vi "assignment4.vi"() -> ()   [LabVIEW 2020]
panel:
  in  "Lower Cut-Off":dbl=30.0
  out "-3db  point":dbl=29.59150674433556
  out "XY Graph":cluster{i32, dbl}[](graph)=[{0, -3.0576747821188574e-08}, {1, -6.013728431780247e-07}, {2, -4.387539160816041e-06}, {3, 3.5095275010031514e-05}, {4, -9.967196479561105e-05}, {5, -0.0002790200036056059}, {6, 0.0011235149369299283}, {7, 0.001968581295715452}, {8, 0.000646352615420884}, {9, -0.0035665225984870207}, {10, -0.010539479788425375}, {11, -0.017748779017499362}, {12, -0.028426417413518115}, {13, -0.044156999314381426}, {14, -0.06675516657396055}, {15, -0.09841418213321976}, {16, -0.14139245078033086}, {17, -0.19793797481989572}, {18, -0.27157149734632635}, {19, -0.36557922218263733}, {20, -0.4489491833896813}, {21, -0.5558693293864396}, {22, -0.7148632709887328}, {23, -0.9010359791461806}, {24, -1.1179952654437506}, {25, -1.3703953898872534}, {26, -1.6597556218137142}, {27, -1.9858590320404002}, {28, -2.348495319765153}, {29, -2.745860990601728}, {30, -3.1755078405015484}, {31, -3.6338601009569373}, {32, -4.117814928392555}, {33, -4.623162452023611}, {34, -5.146444624309847}, {35, -5.683763470785429}, {36, -6.23144744610925}, {37, -6.786719315566659}, {38, -7.346502587344456}, {39, -7.90842063335817}, {40, -8.470649778077558}, {41, -9.03113712355663}, {42, -9.588761700267254}, {43, -10.134599451716804}, {44, -10.67333872530238}, {45, -11.206703608600378}, {46, -11.733812394204042}, {47, -12.252397753569275}, {48, -12.762929323776763}, {49, -13.266641370261848}]
  in  "frequency start":i32
  in  "frequency end":i32=50
  out "?":dynamicdata(graph)=[{"t0"=timestamp(3 s since 1904-01-01), "dt"=0.0001, "Y"=array[1000 elements], "attributes"=variant("NI_ChannelName"=variant(string "Sine_input"), "NI_ExpIsRelativeTime"=variant(bool TRUE), "NI_ExpStartTimeStamp"=variant(timestamp timestamp(3675059466.168606 s since 1904-01-01)), "NI_ExpTimeStamp"=variant(timestamp timestamp(3675059469.168606 s since 1904-01-01)), "NI_ExpXDimension"=variant(string "t"))}]
  in  "stop":bool
  out "Waveform Chart 2":dynamicdata(graph)=[{"t0"=timestamp(3 s since 1904-01-01), "dt"=0.0001, "Y"=array[1000 elements], "attributes"=variant("NI_ChannelName"=variant(string "Sine_input (Filtered)"), "NI_ExpIsRelativeTime"=variant(bool TRUE), "NI_ExpStartTimeStamp"=variant(timestamp timestamp(3675059466.168606 s since 1904-01-01)), "NI_ExpTimeStamp"=variant(timestamp timestamp(3675059469.168606 s since 1904-01-01)), "NI_ExpXDimension"=variant(string "t"), "NI_OriginalChannelName"=variant(string "Sine_input"))}]
  in  "Signal frequency":dbl=30.0
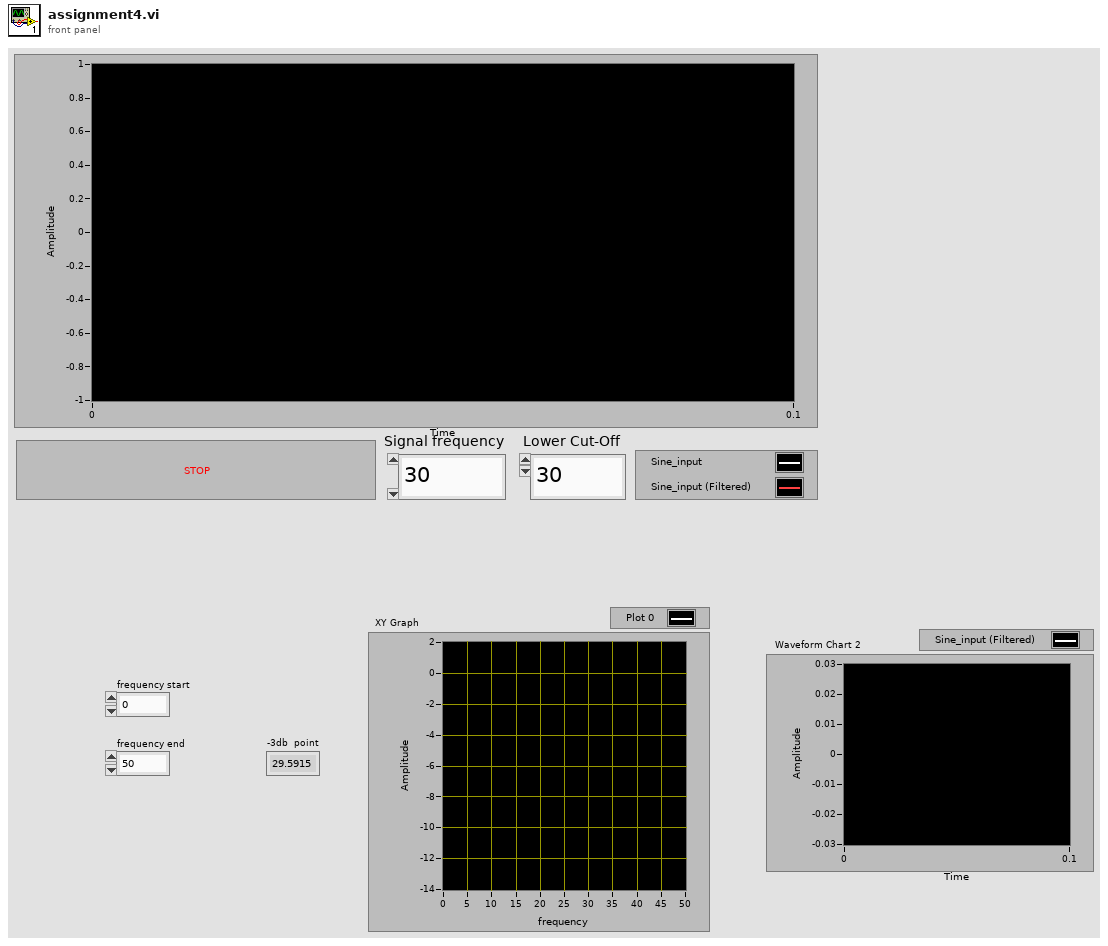
[diagram p1: front panel]
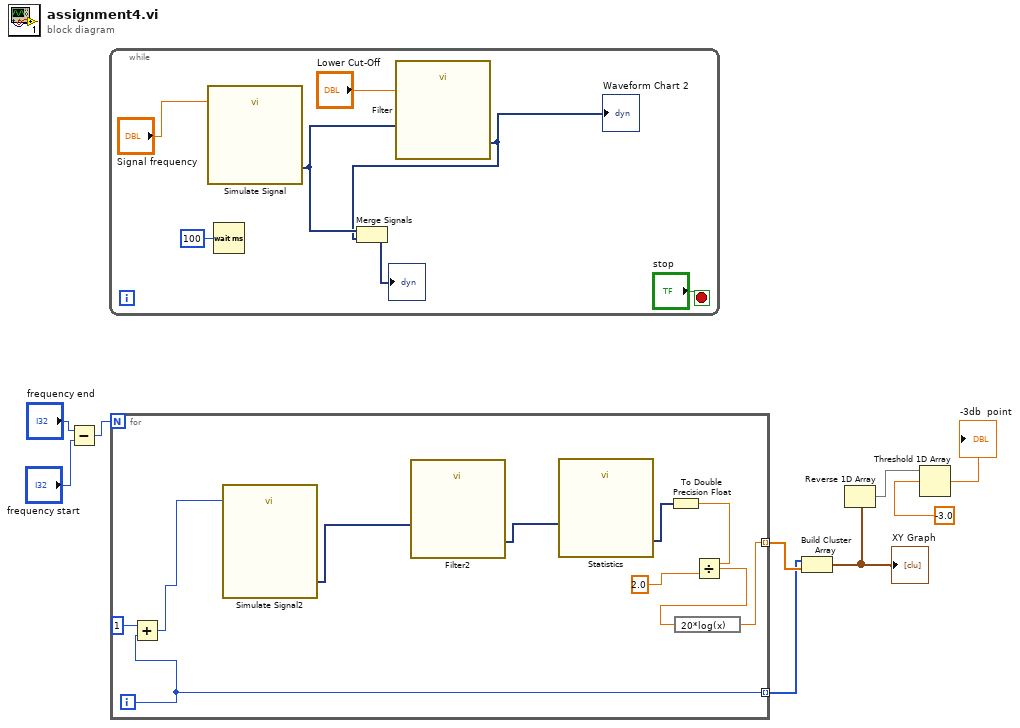
[diagram p0: block diagram]
diagram:
  n1 = Subtract(x="frequency end", y="frequency start") -> (x-y=w7:i32)
  n2 = while {
    stop <- "stop" stop-if-true
    n3 = call "Simulate Signal"("Frequency"="Signal frequency") -> ("Sine_input"=w13:dynamicdata)  [unwired: 13 in, 1 out]
    n4 = Wait (ms)(milliseconds to wait=u32 100) -> ()  [unwired: 1 out]
    n5 = call "Filter"("Lower Cut-Off"="Lower Cut-Off", "Signal"=w13) -> ("Filtered Signal"=w11:dynamicdata)  [unwired: 8 in, 1 out]
    "Waveform Chart 2" <- w11
    n6 = Merge Signals(w13, w11) -> (→"?":dynamicdata)
  }
  n7 = for {
    N: w7 -> [_]
    tunnel: [w17] -> w6 mode=indexing
    tunnel: [w21] -> w5 mode=indexing
    i -> [w21]
    n8 = Add(x=1, y=w21) -> (x+y=w20:i32)
    n9 = call "Simulate Signal2"("Frequency"=w20) -> ("Sine_input"=w26:dynamicdata)  [unwired: 13 in, 1 out]
    n10 = call "Filter2"("Signal"=w26) -> ("Filtered Signal"=w25:dynamicdata)  [unwired: 9 in, 1 out]
    n11 = call "Statistics"("Signals"=w25) -> ("Range"=w23:dynamicdata)  [unwired: 25 in, 1 out]
    n12 = To Double Precision Float(number=w23) -> (double precision float=w22:dbl)
    n13 = Divide(x=w22, y=2.0) -> (x/y=w18:dbl)
    n14 = expression code="20*log(x)"(w18) -> (w17:dbl)
  }
  n15 = Build Cluster Array(w5, w6) -> (w4:cluster{i32, dbl}[])
  "XY Graph" <- w4
  n16 = Reverse 1D Array(array=w4) -> (reversed array=w3:cluster{i32, dbl}[])
  n17 = Threshold 1D Array(2:-3.0 ("threshold y"), 3:w3) -> (0:→"-3db  point":dbl)  [unwired: 1 in]
